vi "ping_2.vi"(0 "Host IP Address":string="127.0.0.1") -> (8 "connected?":bool)   [LabVIEW 2014]
panel:
  out "error out":errorcluster
  out "Execution Time":u32
  out "Status":i32(ring) items=["Success"=0, "DestinationNetworkUnreachable"=11002, "DestinationHostUnreachable"=11003, "DestinationProhibited, DestinationProtocolUnreachable"=11004, "DestinationPortUnreachable"=11005, "NoResources"=11006, "BadOption"=11007, "HardwareError"=11008, "PacketTooBig"=11009, "TimedOut"=11010, "BadRoute"=11012, "TtlExpired"=11013, "TtlReassemblyTimeExceeded"=11014, "ParameterProblem"=11015, "SourceQuench"=11016, "BadDestination"=11018, "DestinationUnreachable"=11040, "TimeExceeded"=11041, "BadHeader"=11042, "UnrecognizedNextHeader"=11043, "IcmpError"=11044, "DestinationScopeMismatch"=11045, "Unknown"=-1]
  in  "timeout":i32=100
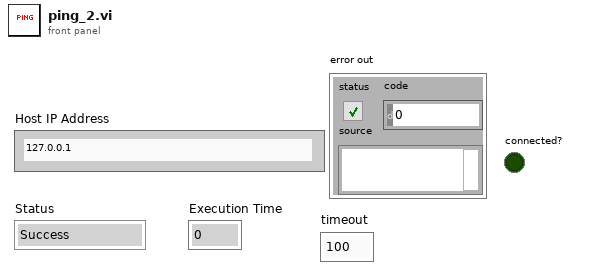
[diagram p1: front panel]
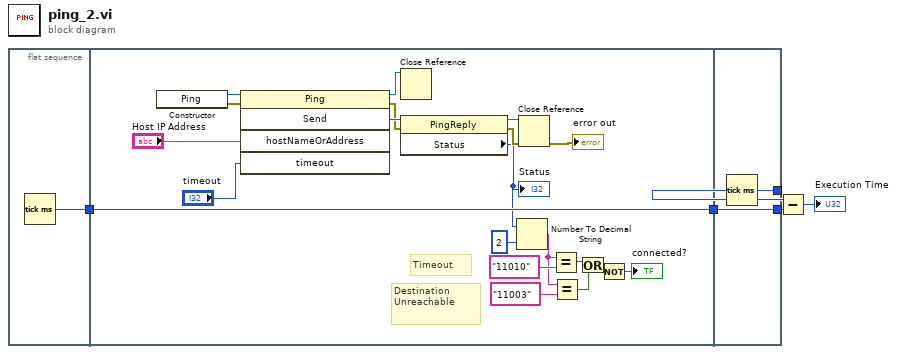
[diagram p0: block diagram]
diagram:
  n1 = flat-sequence {
    tunnel: [w6] -> w5
    tunnel: w5 -> [w20]
    tunnel: [w20] -> w4
    tunnel: [w28] -> w3
    tunnel: w4 -> [w27]
    tunnel: [w27] -> w2
    frame #0 {
      n2 = Tick Count (ms)() -> (millisecond timer value=w6:u32)
    }
    frame #1 {
      # "Destination\nUnreachable"
      # "Timeout"
      n3 = constructor class="Ping"() -> (reference out=w23:refnum<k24>, error out=w18:errorcluster)  [unwired: 3 in, 1 out]
      n4 = invoke class="Ping" method="Send"(reference=w23, error in=w18, "hostNameOrAddress"="Host IP Address", "timeout"="timeout") -> (reference out=w21:refnum<k24>, error out=w19:errorcluster, "Send"=w25:refnum<k24>)  [unwired: 1 in, 2 out]
      n5 = Close Reference(reference=w21) -> ()  [unwired: 1 in, 1 out]
      n6 = property class="PingReply"(reference=w25, error in=w19) -> (reference out=w22:refnum<k24>, error out=w17:errorcluster, "Status"=w15:i32)
      "Status" <- w15
      n7 = Number To Decimal String(number=w15, width (-)=i16 2) -> (decimal integer string=w10:string)
      n8 = Close Reference(reference=w22, error in (no error)=w17) -> (error out=→"error out":errorcluster)
      n9 = Equal?(x=w10, y="11010") -> (x = y?=w12:bool)
      n10 = Equal?(x=w10, y="11003") -> (x = y?=w11:bool)
      n11 = Or(x=w12, y=w11) -> (x .or. y?=w8:bool)
      n12 = Not(x=w8) -> (.not. x?=→"connected?":bool)
    }
    frame #2 {
      n13 = Tick Count (ms)() -> (millisecond timer value=w28:u32)
    }
  }
  n14 = Subtract(x=w3, y=w2) -> (x-y=→"Execution Time":u32)
